vi "Manage Zip Files.vi"(6 "Error Message in":string, 8 "Error In":errorcluster, 11 "Number of copies to keep":i32=5) -> (0 "Error Out":errorcluster, 4 "Error Message out":string)   [LabVIEW 2019]
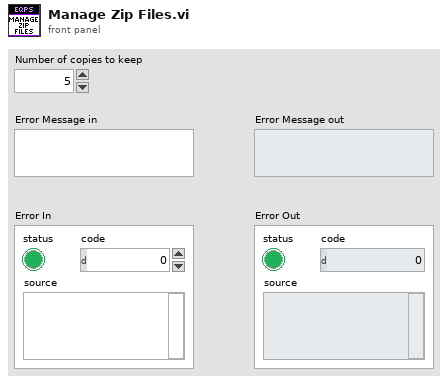
[diagram p1: front panel]
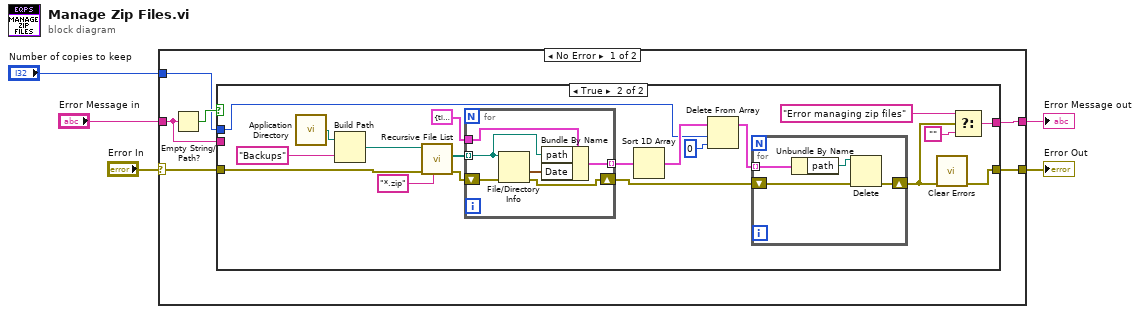
[diagram p0: block diagram]
diagram:
  n1 = case shown="No Error" "Error In" {
    selector: "Error In" -> [w7 w44]
    tunnel: [w8 w44] -> w4
    tunnel: [w10 w43] -> w3
    tunnel: "Error Message in" -> [w9 w43]
    tunnel: "Number of copies to keep" -> [w6 _]
    frame No Error {
      n2 = Empty String/Path?(string/path=w9) -> (empty?=w11:bool)
      n3 = case shown="True" w11 {
        tunnel: [w13 w24] -> w10
        tunnel: w9 -> [w13 _]
        tunnel: [w12 w27] -> w8
        tunnel: w7 -> [w12 w30]
        tunnel: w6 -> [_ w14]
        frame False {
        }
        frame True {
          n4 = call <vilib>:"Application Directory.vi"() -> ("Application Directory"=w31:path)
          n5 = Build Path(base path=w31, name or relative path="Backups") -> (appended path=w29:path)
          n6 = call <vilib>:"Recursive File List.vi"("pattern"="*.zip", "error in (no error)"=w30, "Folder Path"=w29) -> ("error out"=w23:errorcluster, "All Files in Dir"=w22:path[])  [unwired: 4 in, 3 out]
          n7 = for {
            shift-right: [w41] -> w18
            shift-left: w23 -> [w42]
            tunnel: w22 -> [w39] mode=indexing
            tunnel: cluster{"Date":timestamp, "path":path} {"Date"=timestamp(0 s since 1904-01-01), "path"=path ""} -> [w38]
            tunnel: [w37] -> w15 mode=indexing
            n8 = File/Directory Info(path=w39, error in=w42) -> (last mod=w40:timestamp, error out=w41:errorcluster)  [unwired: 5 out]
            n9 = Bundle By Name(cluster=w38, "path"=w39, "Date"=w40) -> (w37:cluster{"Date":timestamp, "path":path})
          }
          n10 = Sort 1D Array(array=w15) -> (sorted array=w21:cluster{"Date":timestamp, "path":path}[])
          n11 = Delete From Array(array=w21, length=w14, index=0) -> (array with subset deleted=w19:cluster{"Date":timestamp, "path":path}[])  [unwired: 1 out]
          n12 = for {
            tunnel: w19 -> [w36] mode=indexing
            shift-right: [w33] -> w17
            shift-left: w18 -> [w35]
            n13 = Unbundle By Name(w36) -> ("path"=w34:path)
            n14 = Delete(path (use dialog)=w34, error in=w35) -> (error out=w33:errorcluster)  [unwired: 3 in, 2 out]
          }
          n15 = call <vilib>:"Clear Errors.vi"("error in (no error)"=w17) -> ("error out"=w27:errorcluster)  [unwired: 5 in, 1 out]
          n16 = Select(t="Error managing zip files", s=w17, f="") -> (s? t:f=w24:string)
        }
      }
    }
    frame Error {
    }
  }
  "Error Out" <- w4
  "Error Message out" <- w3
